vi "ProcessCommand.vi"(5 "Ctl Refnum":refnum<vi>, 7 "Command":variant, 8 "error in (no error)":errorcluster, 9 "Data":T1=variant(string "Default"), 10 "Queue with Cluster Reference":T2, 11 "Internal State Command in":refnum<class "Internal State Command.lvclass">) -> (0 "error out":errorcluster, 2 "Queue (dup)":T2, 3 "Internal State Command out":refnum<class "Internal State Command.lvclass">)   [LabVIEW 2010, in "Internal State Command.lvclass"]
doc: "This VI serves as the dynamic dispatch VI for Internal State Commands.\n\nInputs:\nInternal State Command in - object used for commands within the plugin action loop\n\nCommand - variant data type. \n - not valid in default condition\n - valid as string (for Not A Ref on control reference input)\n\nQueue with Cluster Reference - reference to the EVM queue for inserting commands\n\nCtl Refnum -\n(valid for UserInput Command and Internal State Command objects) \n - UserInput Command - reference to the control that triggered the event; Not A Ref constant allows user defined string constants to be wired to Data input\n - Internal State Command - Not A Ref constant allows user defined string constants to be wired to Data input\n\nData - variant type that whose value can be used to override the control current value being placed in the queue with the command string\n\nerror in - error input cluster\n\nOutputs:\nInternal State Command out - input object passed through\nQueue (dup) - input queue reference passed through\nerror out - error output cluster"
uses:
  Internal State Command.lvclass
  <userlib>/Common/Queue with Cluster/TYP_Queue with Cluster Reference.ctl
  Controls/TYP_VariantDefault.ctl
  Internal State Command.lvclass/Internal State Command.ctl
  <userlib>/Common/Queue with Cluster/Enqueue - ClusterBoth.vi
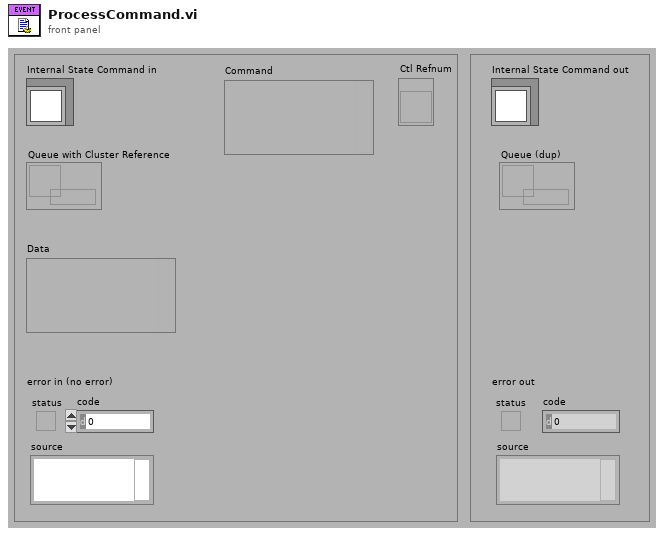
[diagram p1: front panel]
types:
  T1 = typedef "TYP_VariantDefault.ctl" = variant
  T2 = typedef "TYP_Queue with Cluster Reference.ctl" = refnum<queue>
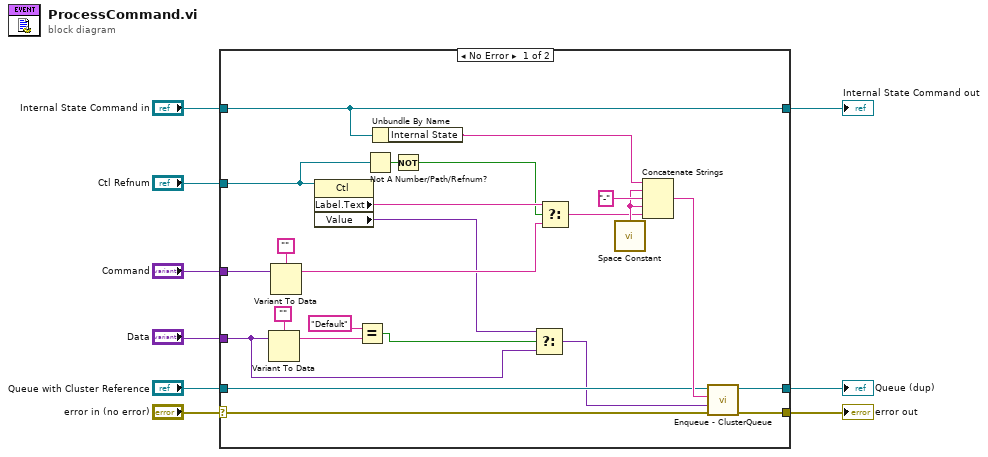
[diagram p0: block diagram]
diagram:
  n1 = case shown="No Error" "error in (no error)" {
    selector: "error in (no error)" -> [w25 w36]
    tunnel: [w26 w36] -> w8
    tunnel: [w20 w35] -> w6
    tunnel: "Internal State Command in" -> [w20 w35]
    tunnel: [w24 w34] -> w5
    tunnel: "Queue with Cluster Reference" -> [w23 w34]
    tunnel: "Command" -> [w21 _]
    tunnel: "Ctl Refnum" -> [w22 _]
    tunnel: "Data" -> [w13 _]
    frame No Error {
      n2 = Variant To Data(Variant=w13, type="") -> (data=w15:string)  [unwired: 1 in, 1 out]
      n3 = Variant To Data(Variant=w21, type="") -> (data=w28:string)  [unwired: 1 in, 1 out]
      n4 = property class="Ctl"(reference=w22) -> ("Label.Text"=w27:string, "Value"=w12:variant)  [unwired: 1 in, 2 out]
      n5 = Equal?(x="Default", y=w15) -> (x = y?=w10:bool)
      n6 = Not A Number/Path/Refnum?(number/path/refnum=w22) -> (NaN/Path/Refnum?=w18:bool)
      n7 = Unbundle By Name(w20) -> ("Internal State"=w19:string)
      n8 = Not(x=w18) -> (.not. x?=w17:bool)
      n9 = Select(t=w12, s=w10, f=w13) -> (s? t:f=w11:T1)
      n10 = Select(t=w27, s=w17, f=w28) -> (s? t:f=w29:string)
      n11 = call <vilib>:"Space Constant.vi"() -> ("String"=w31:string)
      n12 = Concatenate Strings(w19, w31, "-" ("string"), w31, w29) -> (w32:string)
      n13 = call-poly <userlib>:"Enqueue - ClusterQueue.vi"("error in (no error)"=w25, "Data"=w11, "Command"=w32, "Queue with Cluster Reference"=w23) -> ("error out"=w26:errorcluster, "Queue Out (dup)"=w24:T2)  [unwired: 6 in]
    }
    frame Error {
    }
  }
  "error out" <- w8
  "Internal State Command out" <- w6
  "Queue (dup)" <- w5
